vi "Check Data Size.vi"(1 "error in (no error)":errorcluster, 2 "rect":T1, 3 "depth":u8, 4 "flattened image data":u8[](array[numeric])) -> (0 "error out":errorcluster)   [LabVIEW 2020]
doc: "Checks the flattened data to see if the size of the data in bytes is what we expect it to be based on its bounds and depth."
uses:
  Error Cluster From Error Code.vi
  Error Ring.xnode
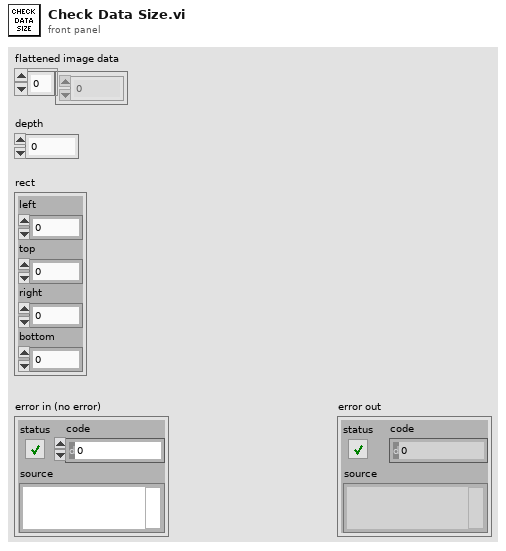
[diagram p1: front panel]
types:
  T1 = cluster{"left":i16, "top":i16, "right":i16, "bottom":i16}
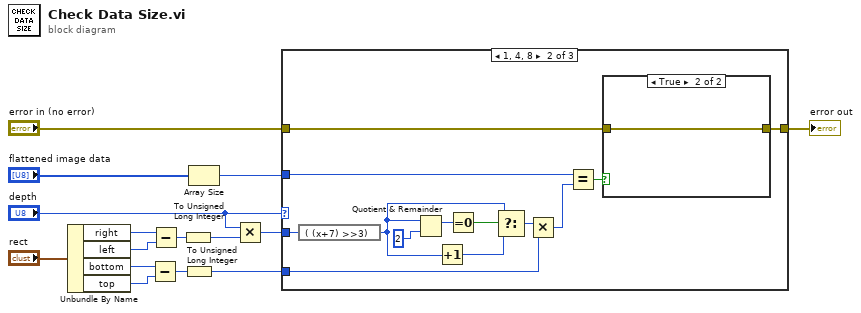
[diagram p0: block diagram]
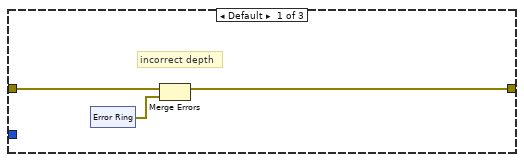
[diagram p2: hidden frame]
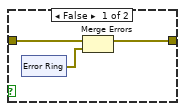
[diagram p3: hidden frame]
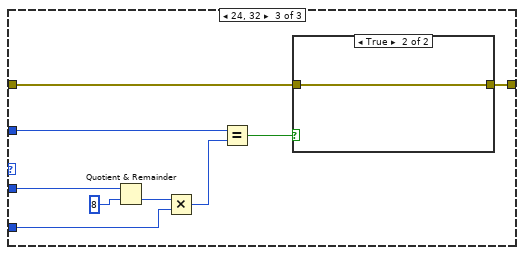
[diagram p4: hidden frame]
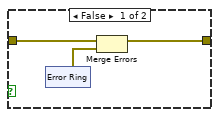
[diagram p5: hidden frame]
diagram:
  n1 = Unbundle By Name("rect") -> ("right"=w8:i16, "left"=w2:i16, "bottom"=w11:i16, "top"=w10:i16)
  n2 = Subtract(x=w11, y=w10) -> (x-y=w13:i16)
  n3 = Subtract(x=w8, y=w2) -> (x-y=w9:i16)
  n4 = To Unsigned Long Integer(number=w9) -> (unsigned 32bit integer=w4:u32)
  n5 = To Unsigned Long Integer(number=w13) -> (unsigned 32bit integer=w3:u32)
  n6 = Array Size(array="flattened image data") -> (size(s)=w15:i32)
  n7 = Multiply(x="depth", y=w4) -> (x*y=w14:u32)
  n8 = case shown="1, 4, 8" "depth" {
    tunnel: "error in (no error)" -> [w18 w30 w50]
    tunnel: [w17 w23 w49] -> w7
    tunnel: w3 -> [_ w33 w46]
    tunnel: w14 -> [_ w32 w48]
    tunnel: w15 -> [_ w31 w52]
    frame Default {
      # "incorrect depth"
      n9 = xnode "Error Ring"() -> ("error out"=w16:errorcluster)
      n10 = Merge Errors(w18, w16) -> (w17:errorcluster)
    }
    frame 1, 4, 8 {
      n11 = expression code="(\t(x+7) >>3)"(w32) -> (w25:u32)
      n12 = Quotient & Remainder(x=w25, y=u32 2 ("x")) -> (x-y*floor(x/y)=w29:u32)  [unwired: 1 out]
      n13 = Increment(x=w25) -> (x+1=w28:u32)
      n14 = Equal To 0?(x=w29) -> (x = 0?=w27:bool)
      n15 = Select(t=w25, s=w27, f=w28) -> (s? t:f=w26:u32)
      n16 = Multiply(x=w26, y=w33) -> (x*y=w35:u32)
      n17 = Equal?(x=w31, y=w35) -> (x = y?=w34:bool)
      n18 = case shown="True" w34 {
        tunnel: w30 -> [w38 w43]
        tunnel: [w37 w43] -> w23
        frame False {
          n19 = xnode "Error Ring"() -> ("error out"=w36:errorcluster)
          n20 = Merge Errors(w38, w36) -> (w37:errorcluster)
        }
        frame True {
        }
      }
    }
    frame 24, 32 {
      n21 = Quotient & Remainder(x=w48, y=u32 8) -> (floor(x/y)=w47:u32)  [unwired: 1 out]
      n22 = Multiply(x=w47, y=w46) -> (x*y=w45:u32)
      n23 = Equal?(x=w52, y=w45) -> (x = y?=w51:bool)
      n24 = case shown="True" w51 {
        tunnel: w50 -> [w55 w60]
        tunnel: [w54 w60] -> w49
        frame False {
          n25 = xnode "Error Ring"() -> ("error out"=w53:errorcluster)
          n26 = Merge Errors(w55, w53) -> (w54:errorcluster)
        }
        frame True {
        }
      }
    }
  }
  "error out" <- w7
